vi "OP600ZP_LaunchLB.vi"(6 "errin":errorcluster, 9 "Application à lancer":path=path "C:/WINDOWS/NOTEPAD.EXE") -> (0 "error out":errorcluster caption="errout")   [LabVIEW 2020]
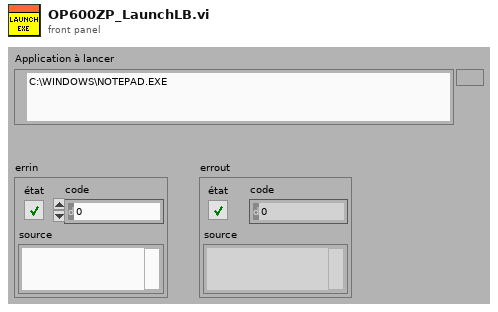
[diagram p1: front panel]
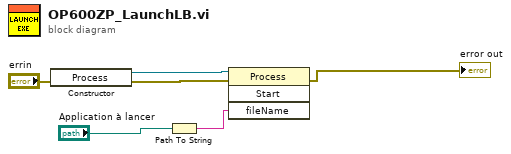
[diagram p0: block diagram]
diagram:
  n1 = constructor class="Process"(error in="errin") -> (reference out=w1:refnum<k24>, error out=w4:errorcluster)  [unwired: 2 in, 1 out]
  n2 = Path To String(path="Application à lancer") -> (string=w3:string)
  n3 = invoke class="Process" method="Start"(reference=w1, error in=w4, "fileName"=w3) -> (error out=→"error out":errorcluster)  [unwired: 1 in, 3 out]
